vi "CRYStep Save Close.vi"(11 "sAction":string) -> ()   [LabVIEW 2013]
uses:
  CRYStepSetup Global.vi
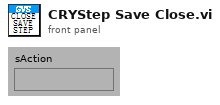
[diagram p1: front panel]
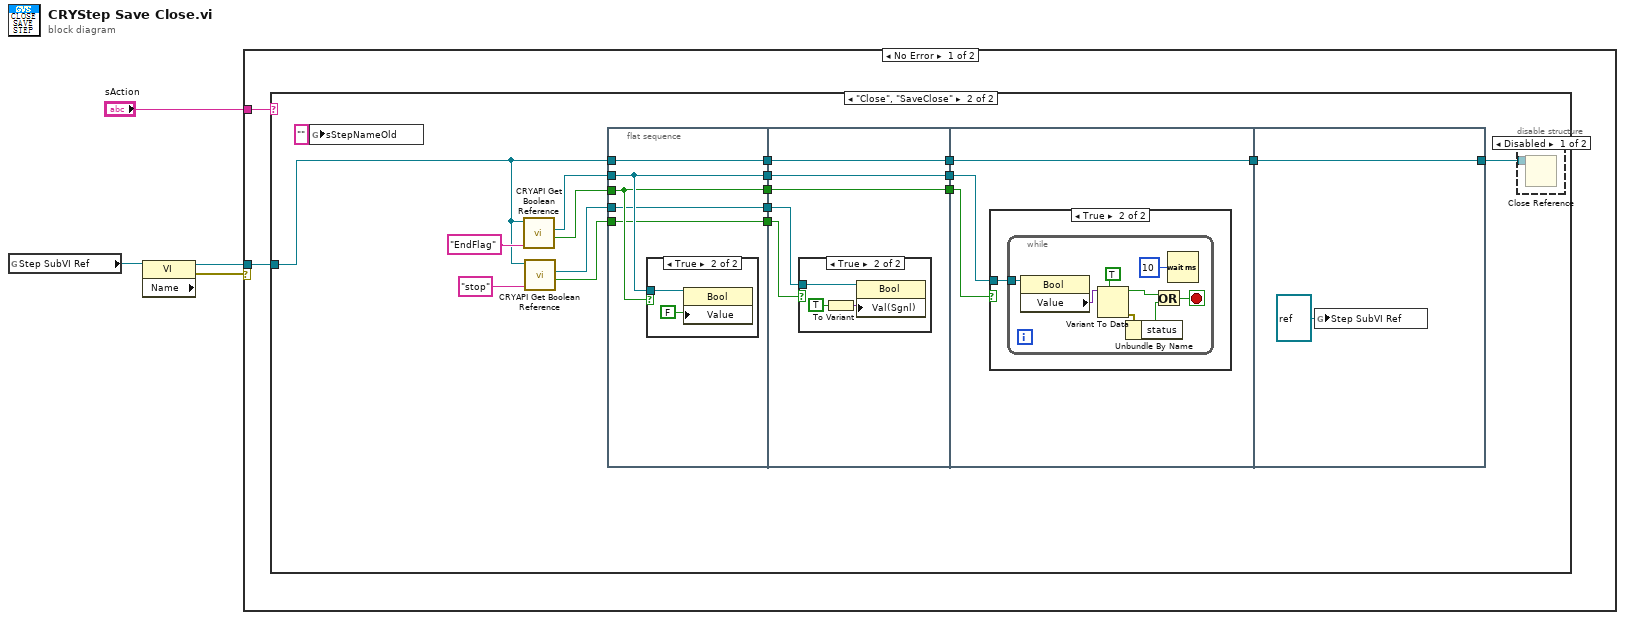
[diagram p0: block diagram]
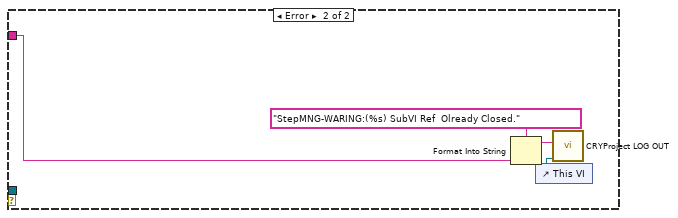
[diagram p7: hidden frame]
diagram:
  n1 = global read "CRYStepSetup Global.vi" "Step SubVI Ref"() -> (w2:refnum<vi>)
  n2 = property class="VI" props=["Name"](reference=w2) -> (reference out=w3:refnum<vi>, error out=w4:errorcluster)  [unwired: 1 in, 1 out]
  n3 = case shown="No Error" w4 {
    tunnel: "sAction" -> [w6 w55]
    tunnel: w3 -> [w5 _]
    frame No Error {
      n4 = case shown="\"Close\", \"SaveClose\"" w6 {
        tunnel: w5 -> [_ w9]
        frame "Save", Default {
          # "??????????????????"
        }
        frame "Close", "SaveClose" {
          n5 = global write "CRYStepSetup Global.vi" "sStepNameOld"("" ("sStepName")) -> ()
          n6 = call "CRYAPI Get Boolean Reference.vi"("Label Name"="EndFlag", "VI Refnum"=w9) -> ("Boolean"=w14:bool, "Boolean Ref"=w13:refnum<vi>)  [unwired: 8 out]
          n7 = call "CRYAPI Get Boolean Reference.vi"("Label Name"="stop", "VI Refnum"=w9) -> ("Boolean"=w11:bool, "Boolean Ref"=w12:refnum<vi>)  [unwired: 8 out]
          n8 = flat-sequence {
            tunnel: w14 -> [w28]
            tunnel: w9 -> [w30]
            tunnel: w13 -> [w29]
            tunnel: w12 -> [w27]
            tunnel: w11 -> [w26]
            tunnel: [w30] -> w24
            tunnel: [w29] -> w23
            tunnel: [w28] -> w22
            tunnel: [w27] -> w21
            tunnel: [w26] -> w20
            tunnel: w24 -> [w35]
            tunnel: w23 -> [w34]
            tunnel: w22 -> [w33]
            tunnel: w21 -> [w36]
            tunnel: w20 -> [w37]
            tunnel: [w35] -> w19
            tunnel: [w34] -> w18
            tunnel: [w33] -> w17
            tunnel: w19 -> [w41]
            tunnel: w18 -> [w42]
            tunnel: w17 -> [w43]
            tunnel: [w41] -> w7
            tunnel: [w54] -> w10
            tunnel: w7 -> [w54]
            frame #0 {
              n9 = case shown="True" w28 {
                tunnel: w29 -> [_ w32]
                frame False {
                }
                frame True {
                  n10 = property class="Bool"(reference=w32, "Value"=FALSE) -> ()  [unwired: 1 in, 2 out]
                }
              }
            }
            frame #1 {
              n11 = case shown="True" w37 {
                tunnel: w36 -> [_ w38]
                frame False {
                }
                frame True {
                  n12 = To Variant(anything=TRUE) -> (Variant=w39:variant)
                  n13 = property class="Bool"(reference=w38, "Val(Sgnl)"=w39) -> ()  [unwired: 1 in, 2 out]
                }
              }
            }
            frame #2 {
              n14 = case shown="True" w43 {
                tunnel: w42 -> [_ w44]
                frame False {
                }
                frame True {
                  n15 = while {
                    tunnel: w44 -> [w52]
                    stop <- w46 stop-if-true
                    n16 = property class="Bool"(reference=w52) -> ("Value"=w51:variant)  [unwired: 1 in, 2 out]
                    n17 = Variant To Data(type=TRUE, Variant=w51) -> (data=w47:bool, error out=w49:errorcluster)  [unwired: 1 in]
                    n18 = Unbundle By Name(w49) -> ("status"=w48:bool)
                    n19 = Or(x=w47, y=w48) -> (x .or. y?=w46:bool)
                    n20 = Wait (ms)(milliseconds to wait=u32 10) -> ()  [unwired: 1 out]
                  }
                }
              }
            }
            frame #3 {
              n21 = global write "CRYStepSetup Global.vi" "Step SubVI Ref"(refnum<vi> refnum ("Step SubVI Ref")) -> ()
            }
          }
          n22 = disable-structure shown="Disabled" {
            disable-tunnel: w10 -> [w25 _]
            frame Disabled {
              n23 = Close Reference(reference=w25) -> ()  [unwired: 1 in, 1 out]
            }
            frame Enabled {
            }
          }
        }
      }
    }
    frame Error {
      n24 = Format Into String(format string="StepMNG-WARING:(%s) SubVI Ref  Olready Closed.", w55) -> (resulting string=w57:string)  [unwired: 2 in, 1 out]
      n25 = control-ref of="This VI"() -> (w58:refnum<vi>)
      n26 = call "CRYProject LOG OUT.vi"("pVIRef"=w58, "sData"=w57) -> ()  [unwired: 10 in]
    }
  }
